vi "Set Finger Forces.vi"(8 "error in (no error)":errorcluster, 10 "Finger Forces":T1={"Thumb"=[82.11798535298313, -180.45157169949402, -21.036974766362523], "Middle"=[216.8568831179214, -112.76947119274729, -2.346783264823202], "Index"=[-13.070660787871816, -94.73788860336559, -5.26647661103047]}, 11 "MF3 in":refnum<class "MF3.lvclass">) -> (0 "error out":errorcluster, 2 "Current setpoints":dbl[](array[numeric]) format="%.2f", 3 "MF3 out":refnum<class "MF3.lvclass">)   [LabVIEW 2011, in "MF3.lvclass"]
uses:
  MF3.lvclass
  controls/Vector3D Fingers.ctl
  controls/Motor Names.ctl
  MF3.lvclass/MF3.ctl
  <vilib>/Analysis/Matrix/Numeric/Multiply/Multiply - RM,RM.vi
  Finger/Finger.lvclass
  <vilib>/Analysis/Matrix/NI_Matrix.lvlib
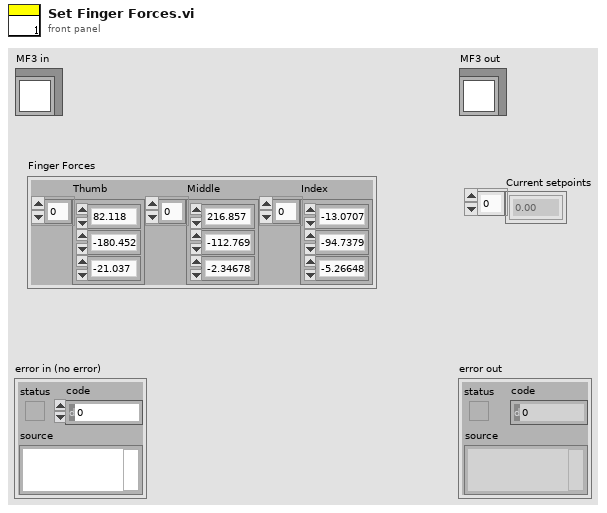
[diagram p1: front panel]
types:
  T1 = typedef "Vector3D Fingers.ctl" = cluster{"Thumb":dbl[], "Middle":dbl[], "Index":dbl[]}
  T2 = typedef "Motor Names.ctl" = enum16{"Thumb1", "Thumb2", "Thumb3", "Middle1", "Middle2", "Middle3", "Redundant", "Index1", "Index2", "Index3"}
  T3 = typedef "NI_Matrix.lvlib/RealMatrix.ctl" = dbl[][]
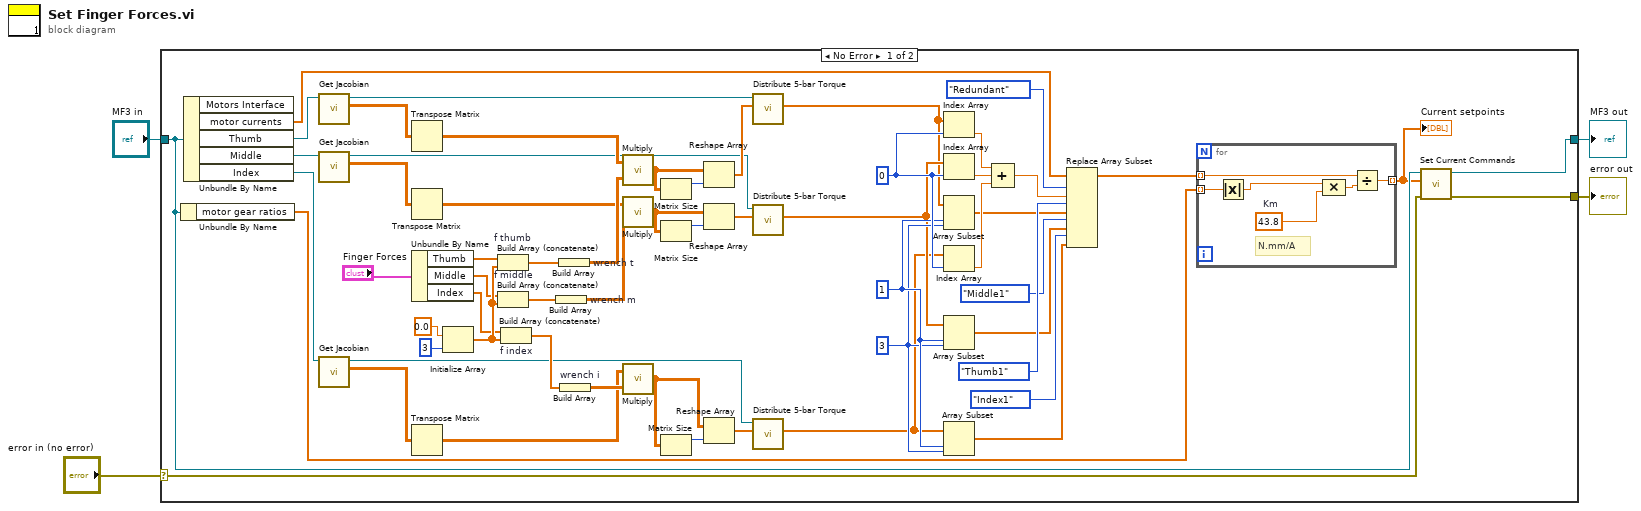
[diagram p0: block diagram]
diagram:
  n1 = case shown="No Error" "error in (no error)" {
    selector: "error in (no error)" -> [w9 w71]
    tunnel: [w8 w71] -> w3
    tunnel: [w7 w70] -> w1
    tunnel: "MF3 in" -> [w10 w70]
    frame No Error {
      w27 = 3 ("length")
      w28 = 1 ("index")
      w32 = 0 ("index")
      n2 = Unbundle By Name(w10) -> ("motor gear ratios"=w15:dbl[])
      n3 = Unbundle By Name(w10) -> ("motor currents"=w20:dbl[], "Thumb"=w63:refnum<class "Finger.lvclass">, "Middle"=w62:refnum<class "Finger.lvclass">, "Index"=w61:refnum<class "Finger.lvclass">)  [unwired: 1 out]
      n4 = call "Get Jacobian.vi"("Finger in"=w63) -> ("Jacobian"=w52:T3, "Finger out"=w36:refnum<class "Finger.lvclass">)  [unwired: 8 in, 1 out]
      n5 = call "Get Jacobian.vi"("Finger in"=w62) -> ("Jacobian"=w53:T3, "Finger out"=w35:refnum<class "Finger.lvclass">)  [unwired: 8 in, 1 out]
      n6 = call "Get Jacobian.vi"("Finger in"=w61) -> ("Jacobian"=w54:T3, "Finger out"=w34:refnum<class "Finger.lvclass">)  [unwired: 8 in, 1 out]
      n7 = Transpose Matrix(1:w52) -> (0:w51:T3)
      n8 = Transpose Matrix(1:w53) -> (0:w49:T3)
      n9 = Unbundle By Name("Finger Forces") -> ("Thumb"=w11:dbl[], "Middle"=w12:dbl[], "Index"=w13:dbl[])
      n10 = Transpose Matrix(1:w54) -> (0:w46:T3)
      n11 = Initialize Array(0.0 ("element"), 3 ("dimension size")) -> (w58:dbl[])
      n12 = Build Array (concatenate) "f thumb"(w11, w58) -> (w57:dbl[])
      n13 = Build Array (concatenate) "f middle"(w12, w58) -> (w56:dbl[])
      n14 = Build Array (concatenate) "f index"(w13, w58) -> (w55:dbl[])
      n15 = Build Array "wrench m"(w56) -> (w48:T3)
      n16 = Build Array "wrench t"(w57) -> (w50:T3)
      n17 = Build Array "wrench i"(w55) -> (w47:T3)
      n18 = call-poly <vilib>:"Multiply.vi"("Real Matrix B"=w50, "Real Matrix A"=w51) -> ("A * B"=w44:T3)
      n19 = call-poly <vilib>:"Multiply.vi"("Real Matrix B"=w48, "Real Matrix A"=w49) -> ("A * B"=w42:T3)
      n20 = call-poly <vilib>:"Multiply.vi"("Real Matrix B"=w47, "Real Matrix A"=w46) -> ("A * B"=w40:T3)
      n21 = Matrix Size(0:w44) -> (1:w45:i32)  [unwired: 1 out]
      n22 = Matrix Size(0:w42) -> (1:w43:i32)  [unwired: 1 out]
      n23 = Matrix Size(0:w40) -> (1:w41:i32)  [unwired: 1 out]
      n24 = Reshape Array(w44, w45) -> (w37:dbl[])
      n25 = Reshape Array(w42, w43) -> (w38:dbl[])
      n26 = Reshape Array(w40, w41) -> (w39:dbl[])
      n27 = call "Distribute 5-bar Torque.vi"("joint_torques"=w37, "Finger in"=w36) -> ("motor_torques"=w24:dbl[])  [unwired: 7 in, 2 out]
      n28 = call "Distribute 5-bar Torque.vi"("joint_torques"=w38, "Finger in"=w35) -> ("motor_torques"=w26:dbl[])  [unwired: 7 in, 2 out]
      n29 = call "Distribute 5-bar Torque.vi"("joint_torques"=w39, "Finger in"=w34) -> ("motor_torques"=w25:dbl[])  [unwired: 7 in, 2 out]
      n30 = Index Array(array=w24, index=w32) -> (element=w33:dbl)
      n31 = Index Array(array=w26, index=w32) -> (element=w30:dbl)
      n32 = Array Subset(array=w24, index=w28, length=w27) -> (w18:dbl[])
      n33 = Index Array(array=w25, index=w32) -> (element=w31:dbl)
      n34 = Array Subset(array=w26, index=w28, length=w27) -> (w17:dbl[])
      n35 = Array Subset(array=w25, index=w28, length=w27) -> (w16:dbl[])
      n36 = Compound Arithmetic op=ADD(w33, w30, w31) -> (w19:dbl)
      n37 = Replace Array Subset "Replace Array Subset"(array=w20, new element #1=w19, index #1=Motor_Names."Redundant" ("Motor Names"), new element #2=w18, index #2=Motor_Names."Thumb1" ("Motor Names"), new element #3=w17, index #3=Motor_Names."Middle1" ("Motor Names"), new element #4=w16, index #4=Motor_Names."Index1" ("Motor Names")) -> (w14:dbl[])
      n38 = for {
        tunnel: w15 -> [w65] mode=indexing
        tunnel: w14 -> [w69] mode=indexing
        tunnel: [w67] -> w6 mode=indexing
        w64 = 43.8  # Km
        # "N.mm/A"
        n39 = Absolute Value(x=w65) -> (abs(x)=w66:dbl)
        n40 = Compound Arithmetic op=MULTIPLY(w66, w64) -> (w68:dbl)
        n41 = Divide(x=w69, y=w68) -> (x/y=w67:dbl)
      }
      "Current setpoints" <- w6
      n42 = call "Set Current Commands.vi"("error in (no error)"=w9, "current commands"=w6, "MF3 in"=w10) -> ("error out"=w8:errorcluster, "MF3 out"=w7:refnum<class "MF3.lvclass">)  [unwired: 7 in]
    }
    frame Error {
    }
  }
  "error out" <- w3
  "MF3 out" <- w1
